vi "5013_Module_configure.vi"() -> ()   [LabVIEW 2010]
uses:
  ADAM Client/Sub VIs/ADAM Controls/Address.ctl
panel:
  in  "Address (Main, Sub reqd.)":T1={"Main"=0, "Ch."=0, "Sub"=0, "Port Name"="MainNetwork"}
  in  "Use checksum":bool
  in  "Range Setting":u16(ring)=3 items=["20     Pt385  -100/100", "21     Pt385  0/100", "22     Pt385  0/200", "23     Pt385  0/600", "24     Pt392 -100/100", "25     Pt392  0/100", "26     Pt392  0/200", "27     Pt392  0/600", "28     Ni392  -80/100", "29     Ni392  0/100"]
  in  "Data Format (ONLY ENG UNITS)":u16(ring) items=["Engineering Units", "% of FSR", "Hex", "Ohms (4013)"]
  in  "Mains Frquency":bool=TRUE
  out "Reply":string
  out "?":string
  # "Happy reply starts \"!\"\nUnhappy reply starts \"?\""
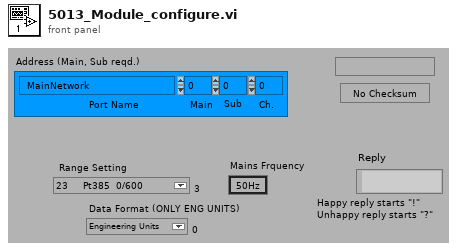
[diagram p1: front panel]
types:
  T1 = typedef "Address.ctl" = cluster{"Main":i32, "Ch.":i32, "Sub":i32, "Port Name":string}
  T2 = cluster{"Boolean array[0]":bool, "Boolean array[1]":bool}
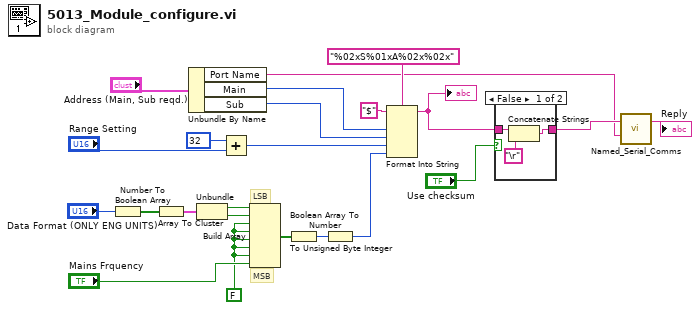
[diagram p0: block diagram]
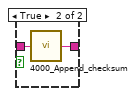
[diagram p2: hidden frame]
diagram:
  w7 = FALSE
  # "MSB"
  # "LSB"
  n1 = Number To Boolean Array(number="Data Format (ONLY ENG UNITS)") -> (Boolean array=w15:bool[])
  n2 = Array To Cluster(array=w15) -> (cluster=w14:T2)
  n3 = Unbundle By Name("Address (Main, Sub reqd.)") -> ("Port Name"=w1:string, "Main"=w6:i32, "Sub"=w5:i32)
  n4 = Unbundle(w14) -> ("Boolean array[0]"=w13:bool, "Boolean array[1]"=w12:bool)
  n5 = Add(x=u16 32, y="Range Setting") -> (x+y=w3:u16)
  n6 = Build Array(w13, w12, w7, w7, w7, w7, w7, "Mains Frquency") -> (w21:bool[])
  n7 = Boolean Array To Number(Boolean array=w21) -> (number=w20:u32)
  n8 = To Unsigned Byte Integer(number=w20) -> (unsigned 8bit integer=w4:u8)
  n9 = Format Into String(format string="%02xS%01xA%02x%02x", initial string="$", w6, w5, w3, w4) -> (resulting string=w19:string)  [unwired: 1 in, 1 out]
  "?" <- w19
  n10 = case shown="False" "Use checksum" {
    tunnel: w19 -> [w26 w28]
    tunnel: [w25 w27] -> w10
    frame False {
      n11 = Concatenate Strings(w26, "\r") -> (w25:string)
    }
    frame True {
      n12 = call "4000_Append_checksum.vi"("ADAM command"=w28) -> ("ADAM string to send"=w27:string)
    }
  }
  n13 = call "Named_Serial_Comms.vi"("Write String"=w10, "Port Name"=w1) -> ("Read"=→"Reply":string)  [unwired: 10 in, 3 out]
